vi "test_property_node.vi"() -> ()   [LabVIEW 2021]
uses:
  Child/Child.lvclass
  Parent/Parent.lvclass/Parent.ctl
  Child/Child.lvclass/Child.ctl
  Parent/Write code.vi
  Child/Write code1.vi
  Parent/Read code.vi
  Child/Read code1.vi
panel:
  out "code1":dbl
  out "message":string
  out "code":dbl
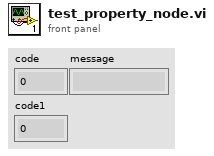
[diagram p1: front panel]
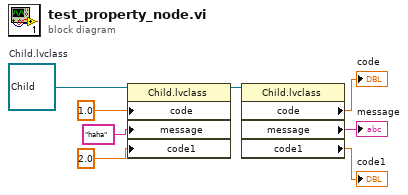
[diagram p0: block diagram]
diagram:
  w8 = refnum<class "Child.lvclass"> refnum  # Child.lvclass
  n1 = property class="Child.lvclass"(reference=w8, "code"=1.0, "message"="haha", "code1"=2.0) -> (reference out=w7:refnum<class "Child.lvclass">)  [unwired: 1 in, 1 out]
  n2 = property class="Child.lvclass"(reference=w7) -> ("code"=→"code":dbl, "message"=→"message":string, "code1"=→"code1":dbl)  [unwired: 1 in, 2 out]
